vi "Controller Process.vi"(8 "error in (no error)":errorcluster, 11 "View Model":T1) -> (0 "error out":errorcluster)   [LabVIEW 2017]
uses:
  View Model/Controls/View Model.ctl
  View Model/Controls/Shared Model.ctl
  Error Handler/Controls/Error Model.ctl
  Error Handler/Controls/Error Data.ctl
  Error Handler/Controls/Error Level.ctl
  Configuration/Controls/Config Model.ctl
  Configuration/Controls/Config Data Record.ctl
  Configuration/Controls/Config Command.ctl
  Controls/Control Model.ctl
  Controls/Elevator Location.ctl
  Controls/Elevator Status.ctl
  Controls/Control Event.ctl
  Controls/Control CMD.ctl
  Controls/Controller - Overhead.ctl
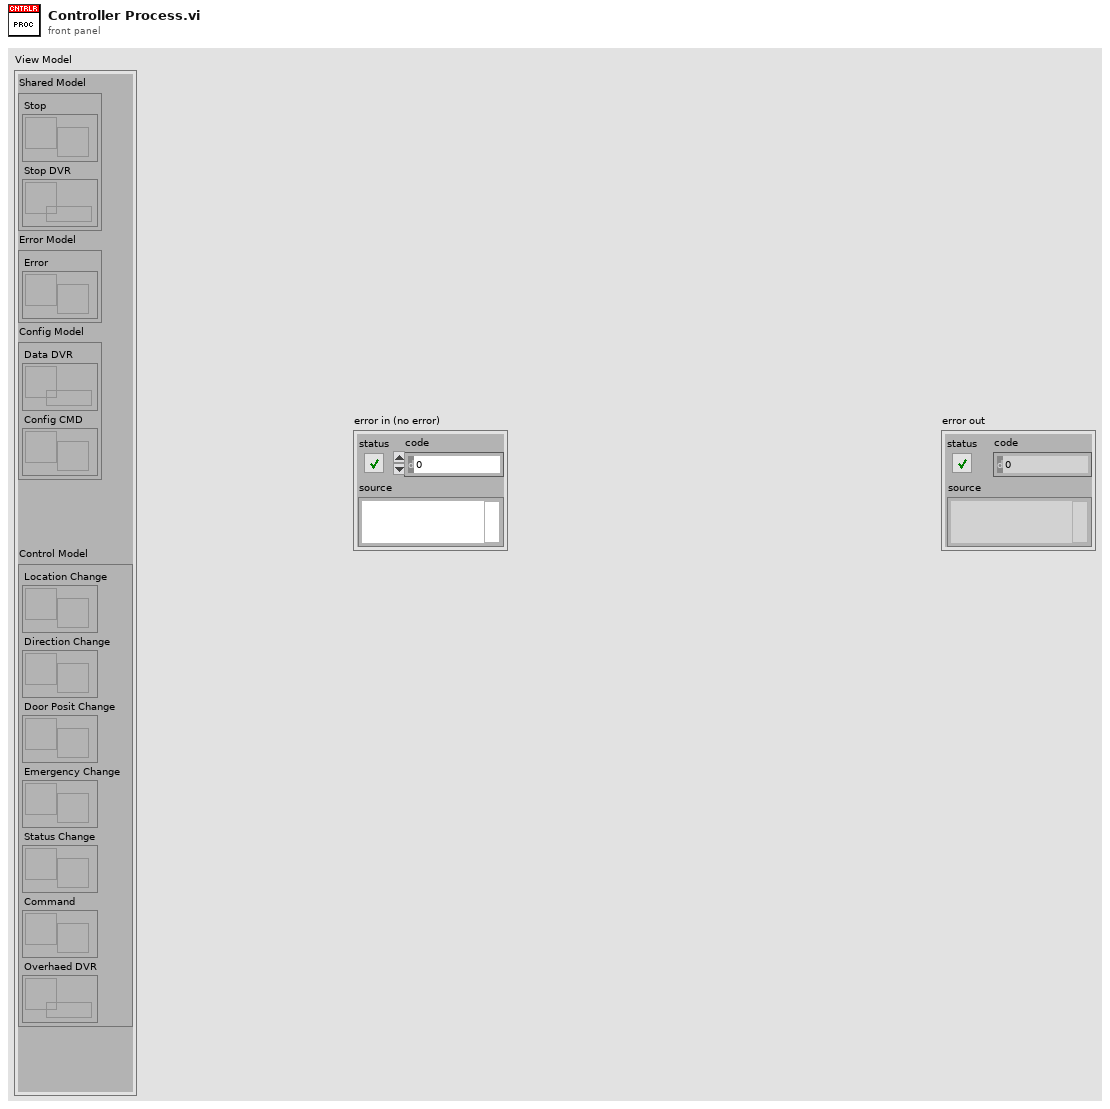
[diagram p1: front panel]
types:
  T1 = typedef "View Model.ctl" = cluster{"Shared Model":T2, "Error Model":T3, "Config Model":T4, "Control Model":T5}
  T2 = typedef "Shared Model.ctl" = cluster{"Stop":refnum<user-event>, "Stop DVR":refnum<data-value>}
  T3 = typedef "Error Model.ctl" = cluster{"Error":refnum<user-event>}
  T4 = typedef "Config Model.ctl" = cluster{"Data DVR":refnum<data-value>, "Config CMD":refnum<user-event>}
  T5 = typedef "Control Model.ctl" = cluster{"Location Change":refnum<user-event>, "Direction Change":refnum<user-event>, "Door Posit Change":refnum<user-event>, "Emergency Change":refnum<user-event>, "Status Change":refnum<user-event>, "Command":refnum<user-event>, "Overhaed DVR":refnum<data-value>}
  T6 = typedef "Config Command.ctl" = enum16{"Read", "Update"}
  T7 = typedef "Elevator Status.ctl" = enum16{"No Request", "Initial", "Wait for 1st Request", "Start and Move", "Continue Move", "Analysis", "Stop at Floor", "Open/Close Door", "Emergency Call", "Terminate"}
  T8 = typedef "Control CMD.ctl" = enum16{"Idle", "Call", "Go Up", "Go Down", "Go to Floor", "Open Door", "Close Door", "Emergency"}
  T9 = typedef "Elevator Location.ctl" = enum16{"1st Floor", "2nd Floor", "3rd Floor", "4th Floor"}
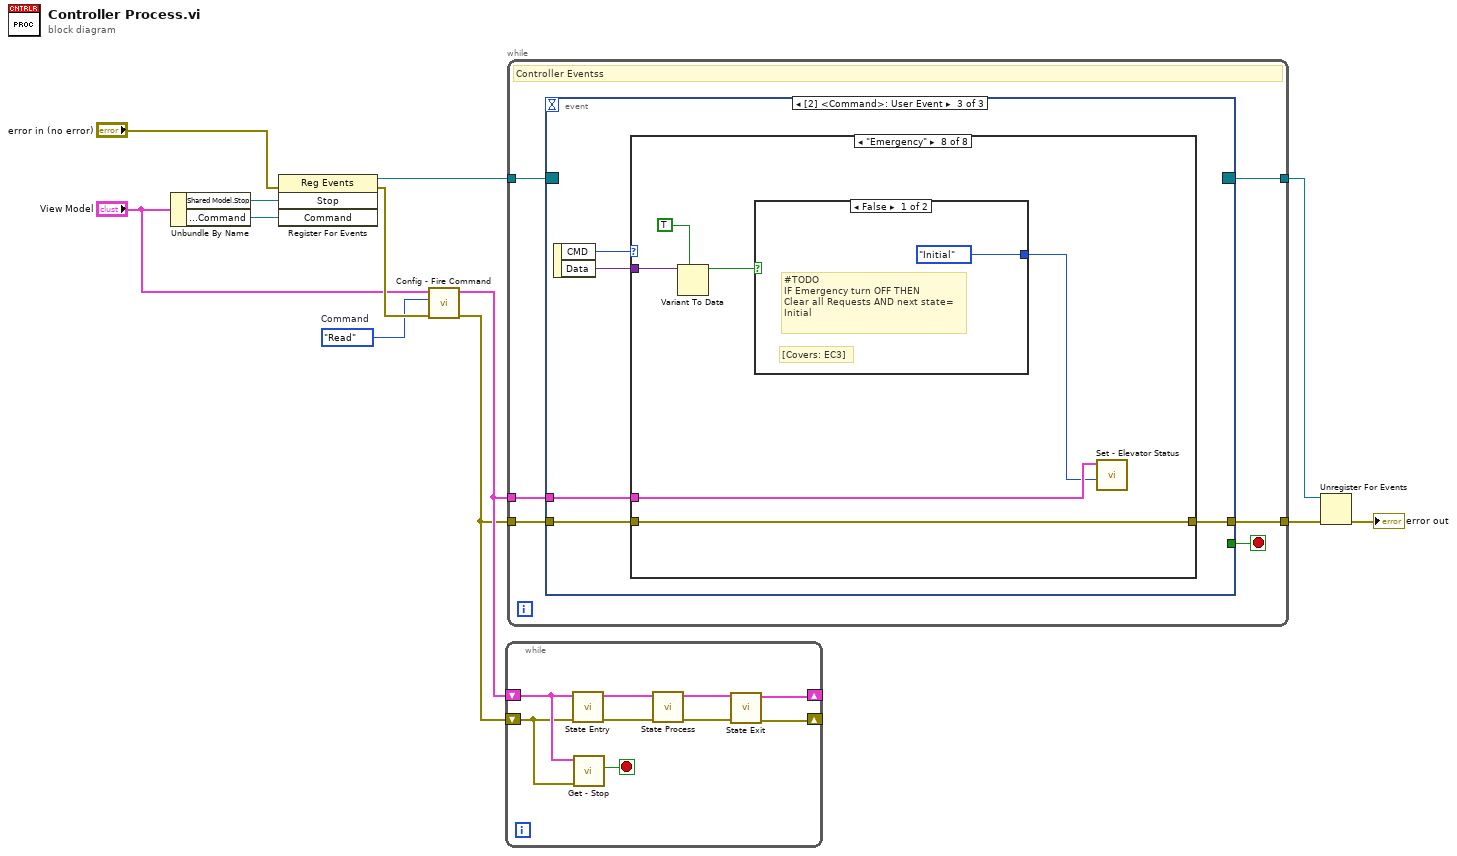
[diagram p0: block diagram]
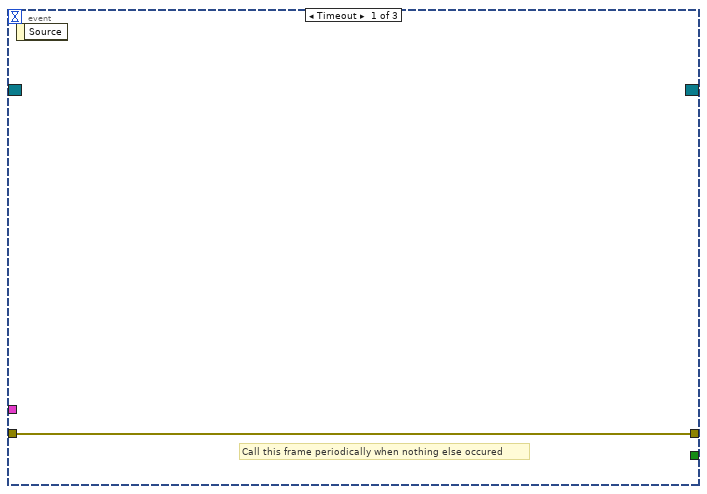
[diagram p2: hidden frame]
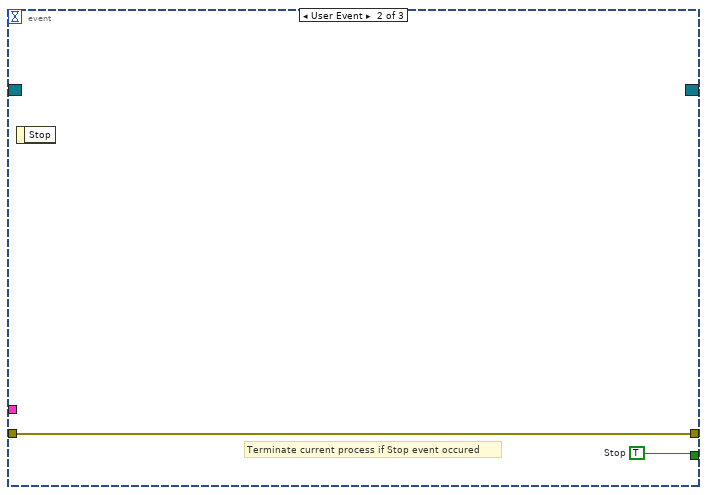
[diagram p3: hidden frame]
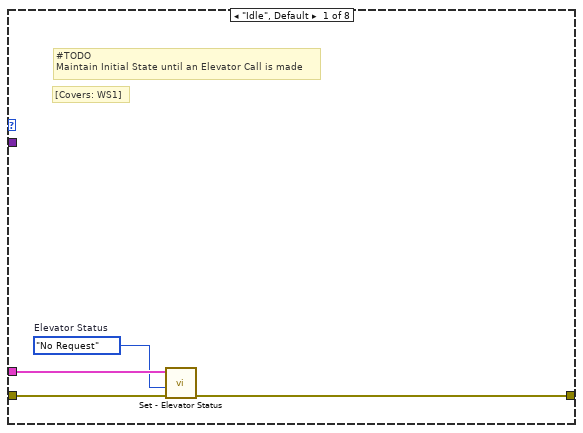
[diagram p4: hidden frame]
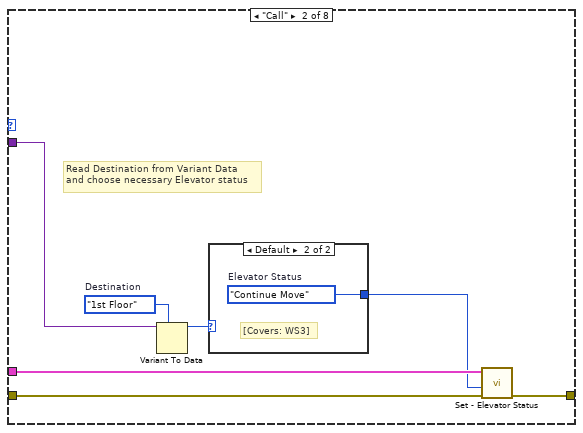
[diagram p5: hidden frame]
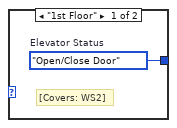
[diagram p6: hidden frame]
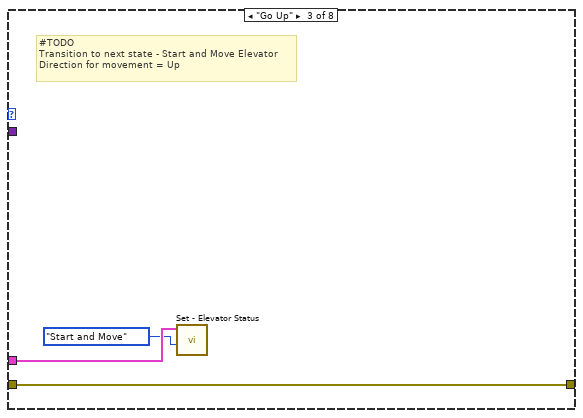
[diagram p7: hidden frame]
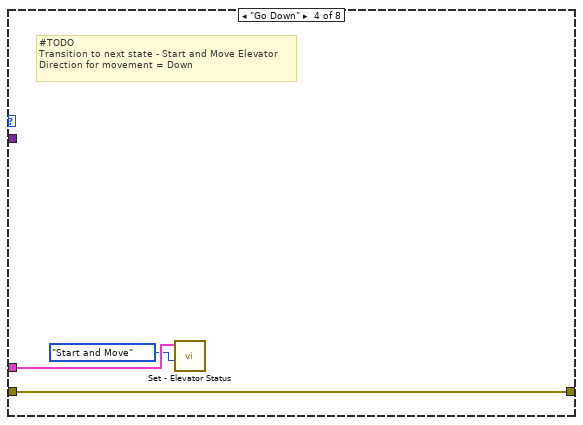
[diagram p8: hidden frame]
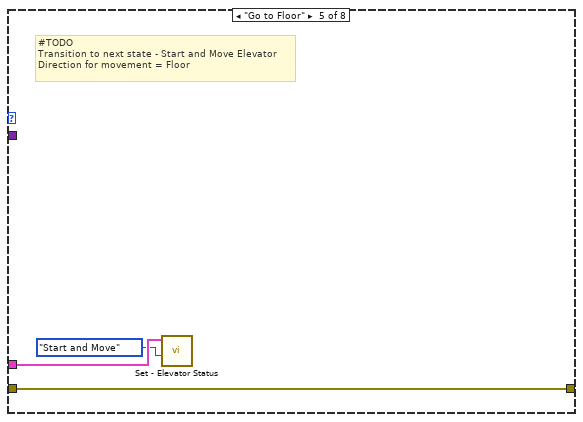
[diagram p9: hidden frame]
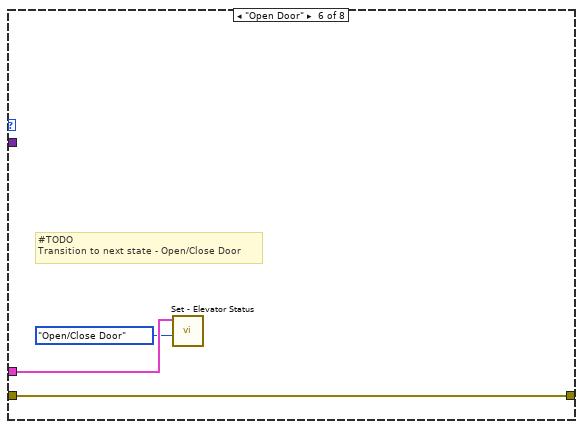
[diagram p10: hidden frame]
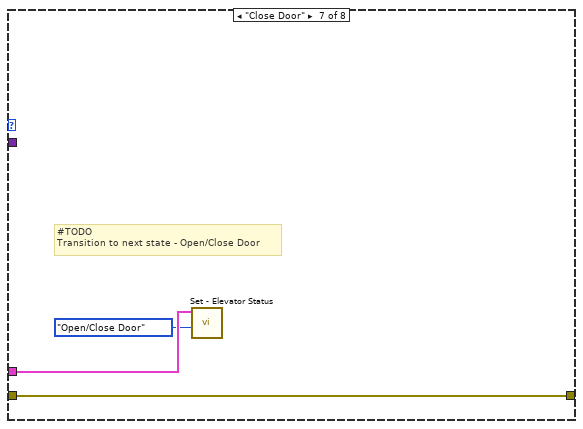
[diagram p11: hidden frame]
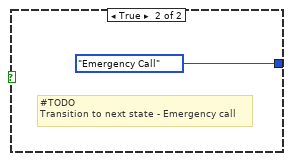
[diagram p12: hidden frame]
diagram:
  w1 = Config_Command."Read"  # Command
  n1 = Unbundle By Name("View Model") -> ("Shared Model.Stop"=w12:refnum<user-event>, "Control Model.Command"=w6:refnum<user-event>)
  n2 = register-events(error in="error in (no error)", w12, w6) -> (reference out=w11:refnum<event-registration>, error out=w5:errorcluster)  [unwired: 1 in]
  n3 = call "Config - Fire Command.vi"("error in (no error)"=w5, "Command"=w1, "View Model"="View Model") -> ("error out"=w2:errorcluster, "View Model"=w3:T1)  [unwired: 7 in]
  n4 = while {
    shift-right: [w14] -> _
    shift-left: w3 -> [w16]
    shift-right: [w13] -> _
    shift-left: w2 -> [w15]
    stop <- w21 stop-if-true
    n5 = call "State Entry.vi"("error in (no error)"=w15, "View Model"=w16) -> ("error out"=w20:errorcluster, "View Model"=w19:T1)  [unwired: 8 in]
    n6 = call "Get - Stop.vi"("error in (no error)"=w15, "View Model"=w16) -> ("Stop"=w21:bool)  [unwired: 7 in, 2 out]
    n7 = call "State Process.vi"("error in (no error)"=w20, "View Model"=w19) -> ("error out"=w18:errorcluster, "View Model"=w17:T1)  [unwired: 8 in]
    n8 = call "State Exit.vi"("error in (no error)"=w18, "View Model"=w17) -> ("error out"=w13:errorcluster, "View Model"=w14:T1)  [unwired: 8 in]
  }
  n9 = while {
    tunnel: w11 -> [w27]
    tunnel: w2 -> [w26]
    tunnel: [w25] -> w8
    tunnel: [w23] -> w9
    tunnel: w3 -> [w22]
    stop <- w24 stop-if-true
    # "Controller Eventss"
    n10 = event shown="[2] <Command>: User Event" {
      selector: w27 -> [_ _ _]
      dyn-events: [_ _ _] -> w23
      timeout: _ -> [_ _ _]
      tunnel: w26 -> [w28 w30 w33]
      tunnel: [w28 w30 w32] -> w25
      tunnel: [_ w29 _] -> w24
      tunnel: w22 -> [_ _ w31]
      event Timeout {
        # "Call this frame periodically when nothing else occured"
        n11 = event-data() -> ()  [unwired: 1 in, 1 out]
      }
      event User Event {
        w29 = TRUE  # Stop
        # "Terminate current process if Stop event occured"
        n12 = event-data() -> ()  [unwired: 1 in, 1 out]
      }
      event User Event {
        n13 = event-data() -> ("CMD"=w35:T8, "Data"=w34:variant)  [unwired: 1 in]
        n14 = case shown="\"Emergency\"" w35 {
          tunnel: w34 -> [_ w46 _ _ _ _ _ w67]
          tunnel: [w38 w43 w51 w54 w57 w60 w63 w69] -> w32
          tunnel: w33 -> [w39 w41 w51 w54 w57 w60 w63 w69]
          tunnel: w31 -> [w37 w42 w50 w53 w56 w59 w62 w68]
          frame "Idle", Default {
            w36 = Elevator_Status."No Request"  # Elevator Status
            # "[Covers: WS1]"
            # "#TODO\nMaintain Initial State until an Elevator Call is made"
            n15 = call "Set - Elevator Status.vi"("error in (no error)"=w39, "Next Status"=w36, "View Model"=w37) -> ("error out"=w38:errorcluster)  [unwired: 7 in, 1 out]
          }
          frame "Call" {
            w45 = Elevator_Location."1st Floor"  # Destination
            # "Read Destination from Variant Data\nand choose necessary Elevator status"
            n16 = Variant To Data(type=w45, Variant=w46) -> (data=w44:T9)  [unwired: 1 in, 1 out]
            n17 = case shown="Default" w44 {
              tunnel: [w47 w48] -> w40
              frame "1st Floor" {
                w47 = Elevator_Status."Open/Close Door"  # Elevator Status
                # "[Covers: WS2]"
              }
              frame Default {
                w48 = Elevator_Status."Continue Move"  # Elevator Status
                # "[Covers: WS3]"
              }
            }
            n18 = call "Set - Elevator Status.vi"("error in (no error)"=w41, "Next Status"=w40, "View Model"=w42) -> ("error out"=w43:errorcluster)  [unwired: 7 in, 1 out]
          }
          frame "Go Up" {
            # "#TODO\nTransition to next state - Start and Move Elevator\nDirection for movement = Up"
            n19 = call "Set - Elevator Status.vi"("Next Status"=Elevator_Status."Start and Move" ("Current Status"), "View Model"=w50) -> ()  [unwired: 8 in, 2 out]
          }
          frame "Go Down" {
            # "#TODO\nTransition to next state - Start and Move Elevator\nDirection for movement = Down"
            n20 = call "Set - Elevator Status.vi"("Next Status"=Elevator_Status."Start and Move" ("Current Status"), "View Model"=w53) -> ()  [unwired: 8 in, 2 out]
          }
          frame "Go to Floor" {
            # "#TODO\nTransition to next state - Start and Move Elevator\nDirection for movement = Floor"
            n21 = call "Set - Elevator Status.vi"("Next Status"=Elevator_Status."Start and Move" ("Current Status"), "View Model"=w56) -> ()  [unwired: 8 in, 2 out]
          }
          frame "Open Door" {
            # "#TODO\nTransition to next state - Open/Close Door"
            n22 = call "Set - Elevator Status.vi"("Next Status"=Elevator_Status."Open/Close Door" ("Current Status"), "View Model"=w59) -> ()  [unwired: 8 in, 2 out]
          }
          frame "Close Door" {
            # "#TODO\nTransition to next state - Open/Close Door"
            n23 = call "Set - Elevator Status.vi"("Next Status"=Elevator_Status."Open/Close Door" ("Current Status"), "View Model"=w62) -> ()  [unwired: 8 in, 2 out]
          }
          frame "Emergency" {
            n24 = Variant To Data(type=TRUE, Variant=w67) -> (data=w65:bool)  [unwired: 1 in, 1 out]
            n25 = case shown="False" w65 {
              tunnel: [Elevator_Status."Initial" ("Current Status") Elevator_Status."Emergency Call" ("Current Status")] -> w64
              frame False {
                # "[Covers: EC3]"
                # "#TODO\nIF Emergency turn OFF THEN\nClear all Requests AND next state=\nInitial"
              }
              frame True {
                # "#TODO\nTransition to next state - Emergency call"
              }
            }
            n26 = call "Set - Elevator Status.vi"("Next Status"=w64, "View Model"=w68) -> ()  [unwired: 8 in, 2 out]
          }
        }
      }
    }
  }
  n27 = Unregister For Events(event registration refnum=w9, error in=w8) -> (error out=→"error out":errorcluster)
